vi "ColorMatch_Setting_UI.vi"(0 "Vision_Image In":T3(plugin-control), 1 "Coord?":bool, 5 "List ROI 2":refnum<vi>, 7 "PreProcess In":T1, 9 "ProjectName":string="CDF", 11 "error in (no error)":errorcluster, 12 "Parameter":string, 14 "RootPath":path) -> (4 "Analysis_Setting":string, 6 "Match Flag":bool[](array[boolean]), 8 "Match Score":i32[](array[numeric]), 10 "Cancel?":bool, 15 "error out":errorcluster)   [LabVIEW 2019]
uses:
  <vilib>/vision/NI_Vision_Development_Module.lvlib
  Controls/Analysis_Setting.ctl
  <vilib>/userdefined/High Color/IMAQdx.ctl
  <vilib>/vision/Image Controls.llb/IMAQ Image.ctl
  Controls/_UI Command Cluster/ColorMatch_UI Command.ctl
  Controls/ColorMatch/Analysis_ColorMatch_Parameter.ctl
  cb7ab341-9881-4345-8d5f-fb9cb1b2a84f.vi
  73ae4806-8b8b-4118-bada-9954a96a792c.vi
  <vilib>/Utility/miscctls.llb/LVPointTypeDef.ctl
  c15c5890-f854-46a2-b98b-929fa5ff6ec0.vi
  76c2e7b3-0f24-4336-b544-f46512082401.vi
  Controls/V_Analysis_Type.ctl
  Ctrl/VisionProcessName.ctl
panel:
  out "PreProcess":T1
  in  "Match Saturation Threshold":i32=80 min=10 max=255 step=1
  out "RunROI":T2
  in  "SetROI":bool
  out "TemplateROI":T2
  out "Template Image":T3(plugin-control)
  in  "Cancel":bool
  in  "Done":bool
  in  "ColorMatchTab":T4(tab)
  in  "Minimum Match Score":dbl=750.0 min=10.0 max=255.0 step=1.0
  in  "Color Sensitivity":u32(ring) items=["Low", "Medium", "High"]
  in  "Learn & Match Saturation Threshold":i32=80 min=10 max=255 step=1
  in  "Vision_Image":T3(plugin-control)
  in  "Run Algorithm":bool
  in  "SetTemplate":bool
  # "Use Ctrl to Select multiple ROI"
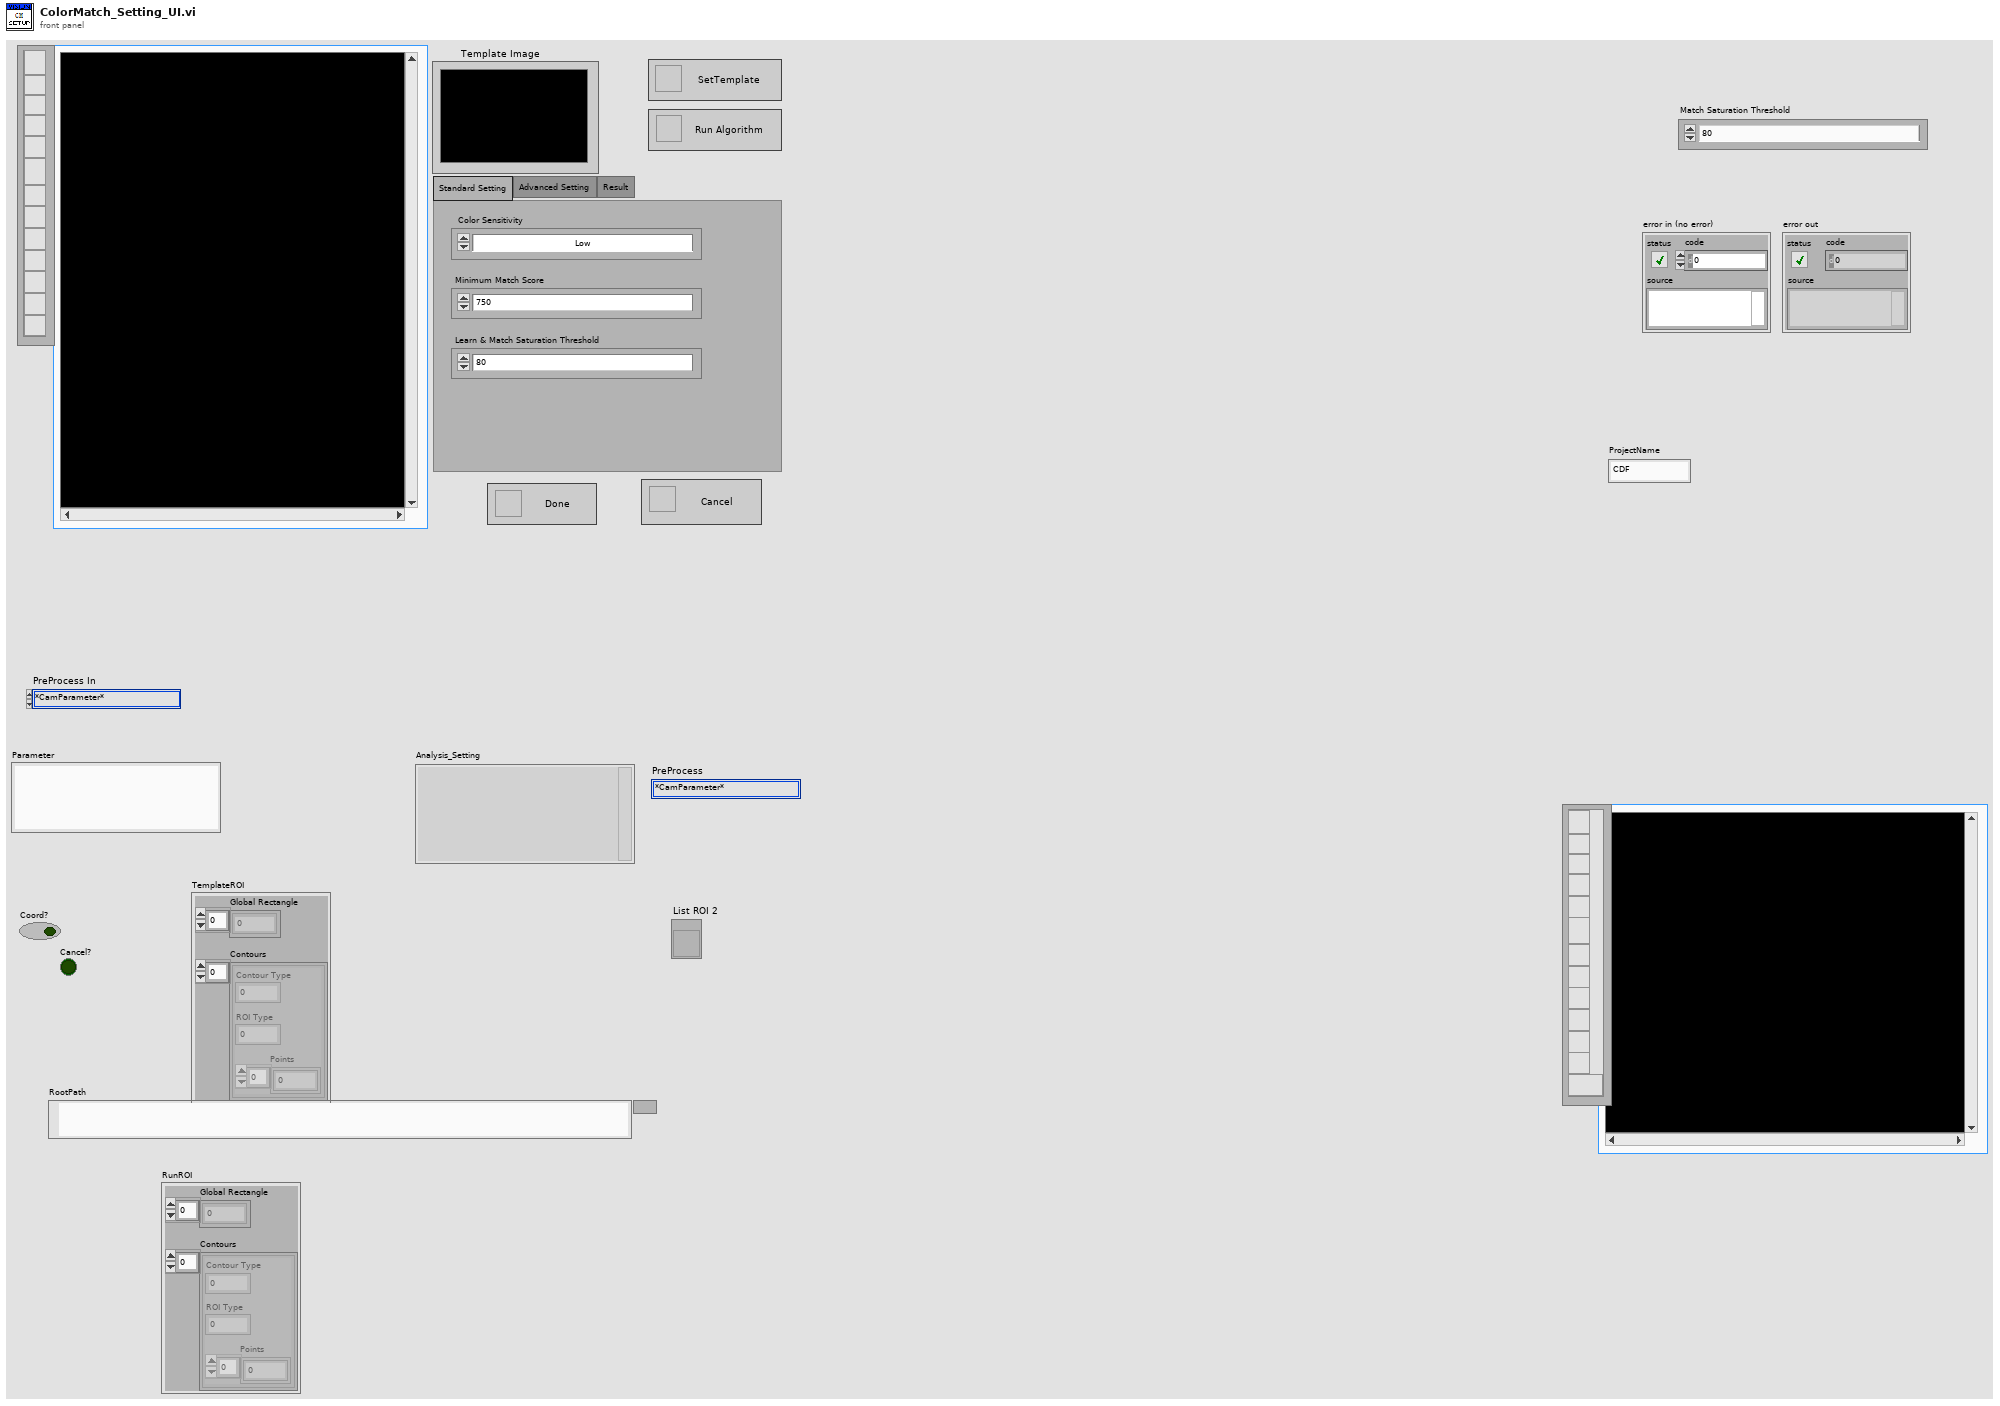
[diagram p1: front panel]
types:
  T1 = typedef "VisionProcessName.ctl" = enum16{"*CamParameter*", "CamAttributes", "*Preprocess*", "CG_Brightness", "C_Plane Extraction", "C_Threshold", "G_Lookup Table", "G_Threshold"}
  T2 = cluster{"Global Rectangle":i32[], "Contours":cluster{"Contour Type":u32, "ROI Type":u32, "Points":i32[]}[]}
  T3 = typedef "IMAQ Image.ctl" = refnum<image>
  T4 = enum32{"Standard Setting", "Advanced Setting", "Result"}
  T5 = typedef "Image Type" = u32
  T6 = typedef "ColorMatch_UI Command.ctl" = enum16{"Init", "Done", "Cancel", "RunAlgorithm", "SetTemplate", "SetROI", "ClearOverlay", "Load Template", "Draw Overlay", "Offset"}
  T7 = typedef "LVPointTypeDef.ctl" = cluster{"Horizontal":i16, "Vertical":i16}
  T8 = typedef "IMAQdx.ctl" = refnum<k21>
  T9 = typedef "Analysis_Setting.ctl" = cluster{"PreProcess":T10, "Parameter":string}
  T10 = typedef "V_Analysis_Type.ctl" = enum16{"None", "C_Color Pattern Matching", "G_PatternMatching", "G_ShapeDectect", "G_GeometricMatch", "B_Area Check"}
  T11 = enum8{"Enabled", "Disabled", "Disabled and Grayed Out"}
  T12 = typedef "Analysis_ColorMatch_Parameter.ctl" = cluster{"Color Sensitivity":u32, "Learn Saturation Threshold":i32, "Minimum Match Score":dbl, "Match Saturation Threshold":i32, "ROI Descriptor":T13, "TemplatePath":string, "ColorSpectrum":dbl[]}
  T13 = typedef "ROI Descriptor" = cluster{"Global Rectangle":i32[], "Contours":cluster{"ID":enum32{"External", "Internal"}, "Type":u32, "Coordinates":i32[]}[]}
  T14 = cluster{"Desired Font (Application)":enum16{"User-specified Font", "Application Font", "System Font", "Dialog Font"}, "[User-specified Font]":cluster{"Font Name":string, "Size":i16, "Strikeout?":bool, "Italic?":bool, "Underline?":bool, "Outline?":bool, "Shadow?":bool, "Bold?":bool, "Rotation Angle":dbl}, "Horizontal Alignment":i16, "Vertical Alignment":i16}
  T15 = cluster{"Contour Type":u32, "ROI Type":u32, "Points":i32[]}
  T16 = cluster{"Position":cluster{"x":sgl, "y":sgl}, "Angle":sgl, "Scale":sgl, "Score":sgl, "Bounding Box":cluster{"x":sgl, "y":sgl}[]}[]
  T17 = cluster{"Contour Type":u32, "ROI Type":u32, "Points":i32[]}[]
  T18 = enum16{"Init", "Done", "Cancel", "RunAlgorithm", "SetTemplate", "SetROI", "ClearOverlay"}
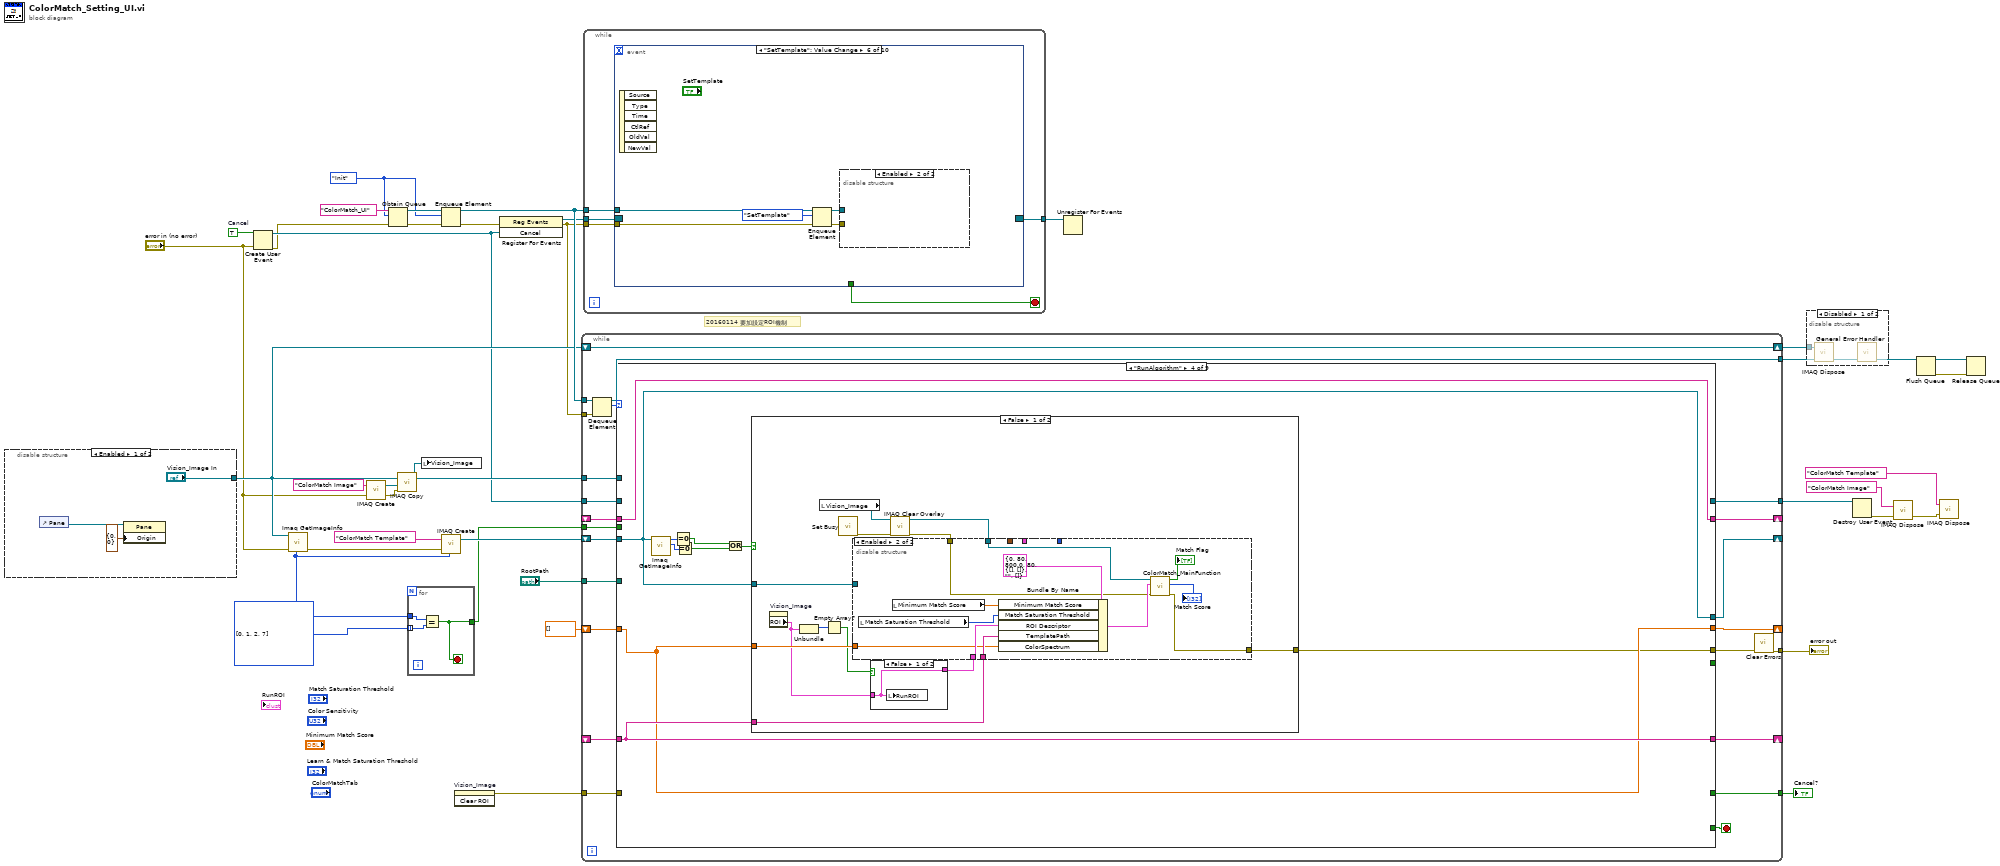
[diagram p0: block diagram]
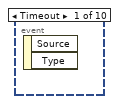
[diagram p2: hidden frame]
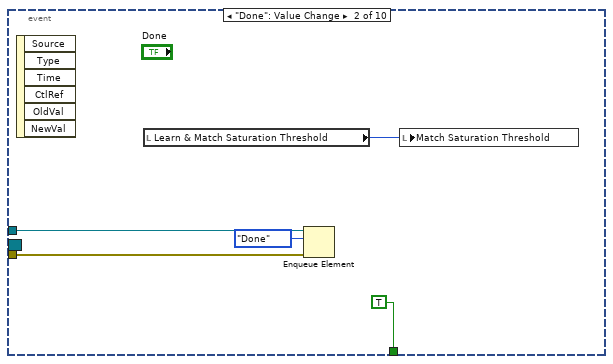
[diagram p3: hidden frame]
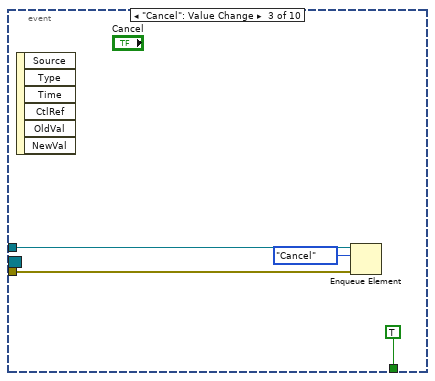
[diagram p4: hidden frame]
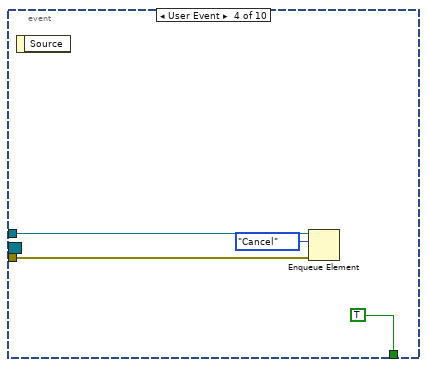
[diagram p5: hidden frame]
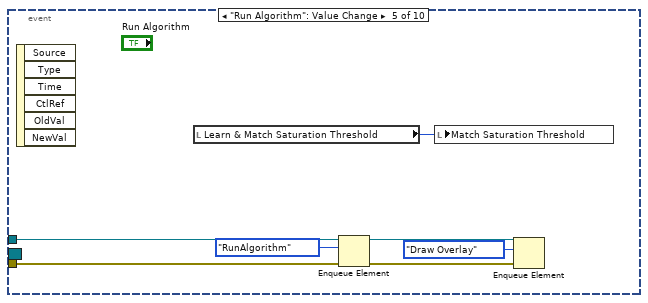
[diagram p6: hidden frame]
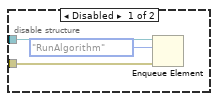
[diagram p7: hidden frame]
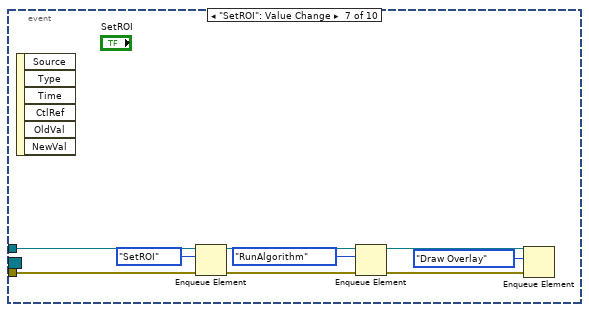
[diagram p8: hidden frame]
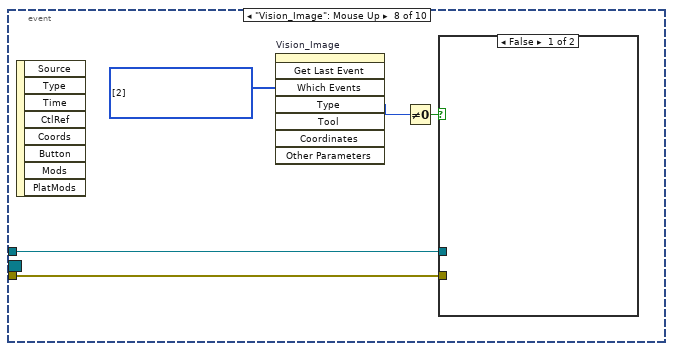
[diagram p9: hidden frame]
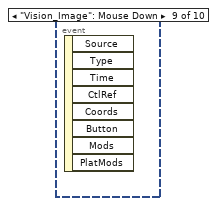
[diagram p11: hidden frame]
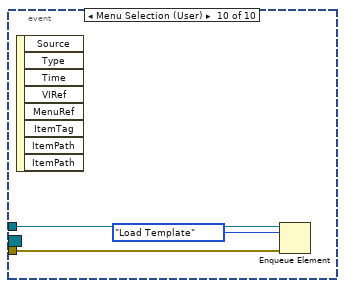
[diagram p12: hidden frame]
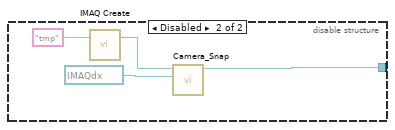
[diagram p13: hidden frame]
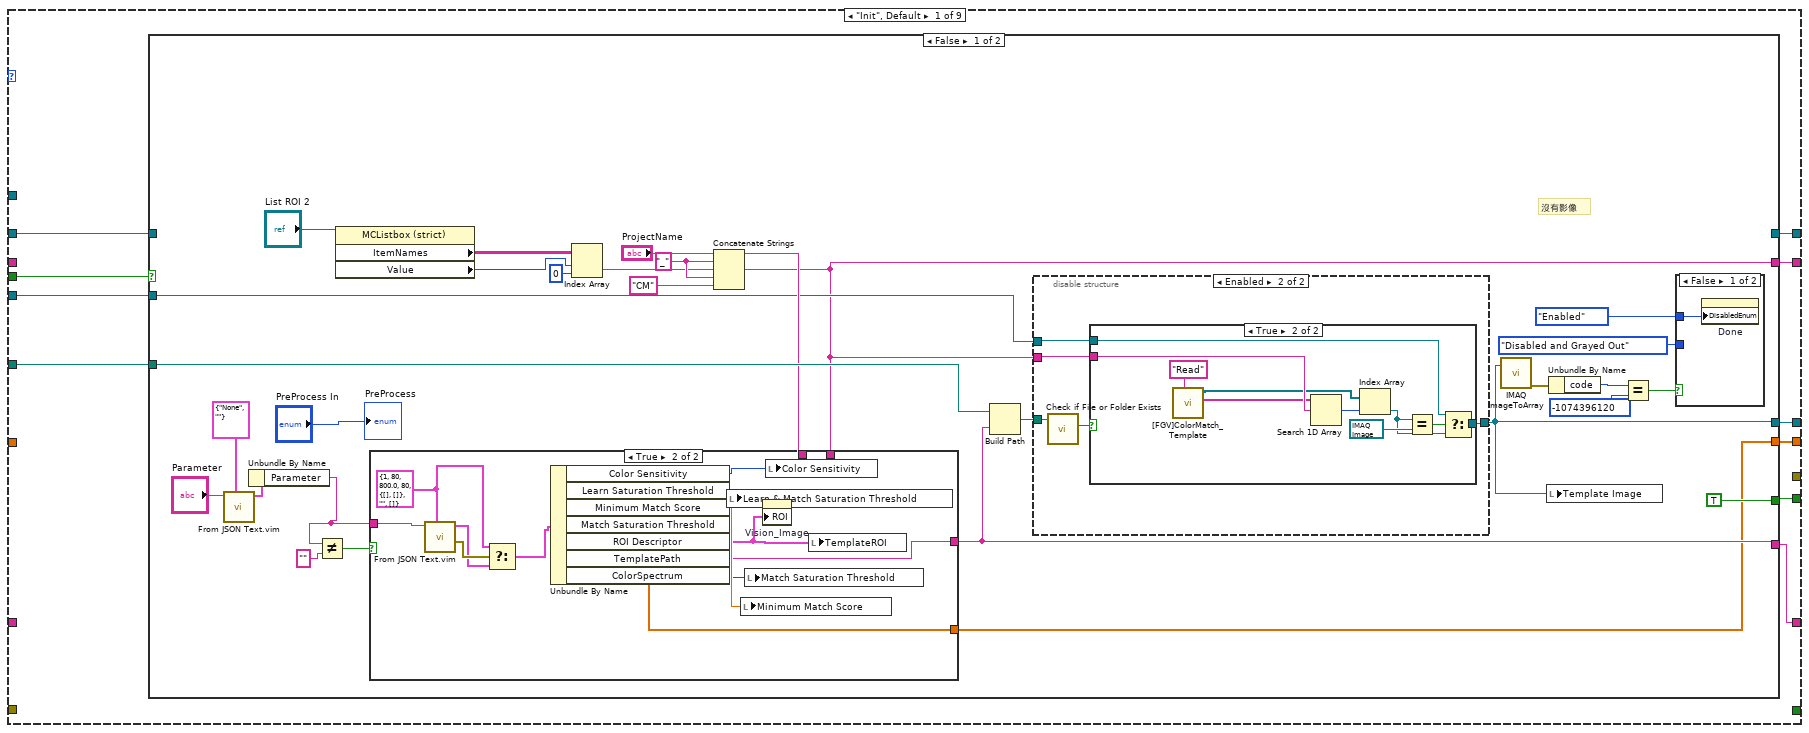
[diagram p15: hidden frame]
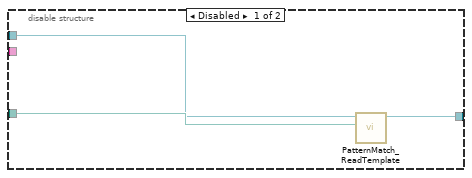
[diagram p16: hidden frame]
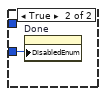
[diagram p18: hidden frame]
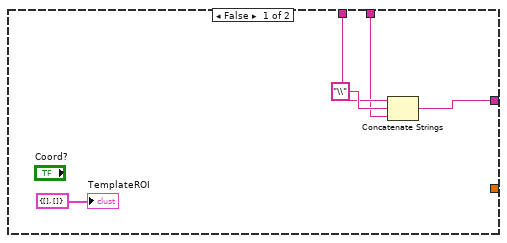
[diagram p19: hidden frame]
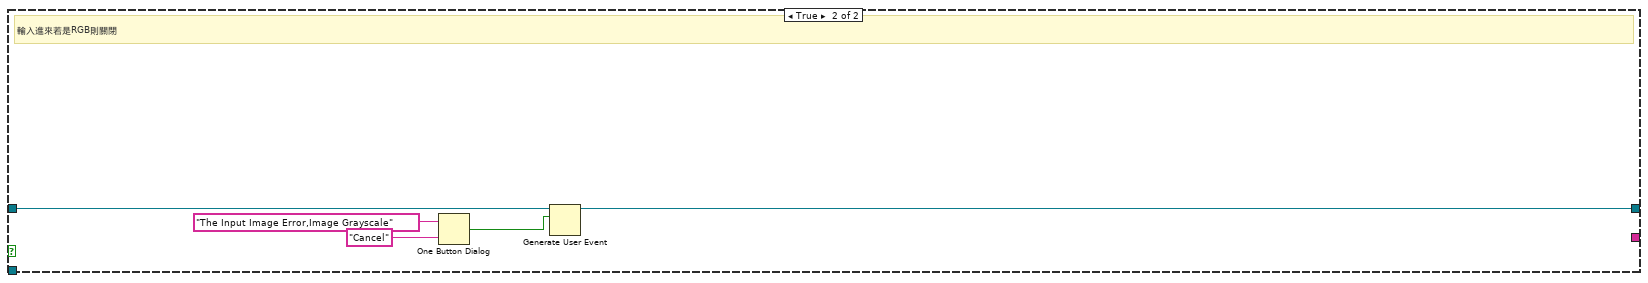
[diagram p20: hidden frame]
diagram:
  w20 = TRUE  # Cancel
  w3 = T5[] [0, 1, 2, 7] items=["Grayscale (U8)", "Grayscale (I16)", "Grayscale (SGL)", "Complex (CSG)", "RGB (U32)", "HSL (U32)", "RGB (U64)", "Grayscale (U16)"] ("x")
  w21 = ColorMatch_UI_Command."Init"
  # "20160114 要加設定ROI機制"
  n1 = disable-structure shown="Enabled" {
    disable-tunnel: ["Vision_Image In" w42] -> w24
    frame Enabled {
      n2 = control-ref of="Pane"() -> (w40:refnum<vi>)
      n3 = property class="Pane"(reference=w40, "Origin"=T7 {"Horizontal"=0, "Vertical"=0}) -> ()  [unwired: 1 in, 2 out]
    }
    frame Disabled {
      n4 = call "IMAQ Create"("Image Name"="tmp") -> ("New Image"=w43:T3)  [unwired: 4 in, 1 out]
      n5 = call "Camera_Snap.vi"("Camera Session In"=T8 "cam0", "Image In"=w43) -> ("New Image"=w42:T3)  [unwired: 8 in, 1 out]
    }
  }
  n6 = Create User Event(user event datatype=w20, error in="error in (no error)") -> (user event=w18:refnum<user-event>, error out=w9:errorcluster)
  n7 = call "Imaq GetImageInfo"("error in (no error)"="error in (no error)", "Image"=w24) -> ("error out"=w7:errorcluster, "Image Type"=w4:T5)  [unwired: 2 in, 6 out]
  n8 = call "IMAQ Create"("Image Name"="ColorMatch Image", "error in (no error)"="error in (no error)") -> ("New Image"=w33:T3, "error out"=w8:errorcluster)  [unwired: 3 in]
  n9 = Obtain Queue(name (unnamed)="ColorMatch_UI", element data type=w21, error in (no error)=w9) -> (queue out=w30:refnum<queue>, error out=w29:errorcluster)  [unwired: 2 in, 1 out]
  n10 = call "IMAQ Copy"("error in (no error)"=w8, "Image Dst"=w33, "Image Src"=w24) -> ("Image Dst Out"=w32:T3)  [unwired: 3 in, 1 out]
  n11 = for {
    tunnel: w4 -> [w48]
    tunnel: w3 -> [w47] mode=indexing
    tunnel: [w46] -> w2
    stop <- w46 stop-if-true
    n12 = Equal?(x=w48, y=w47) -> (x = y?=w46:bool)
  }
  n13 = local write "Vision_Image"(w32) -> ()
  n14 = Enqueue Element(queue=w30, element=w21, error in (no error)=w29) -> (queue out=w26:refnum<queue>, error out=w15:errorcluster)  [unwired: 1 in, 1 out]
  n15 = call "IMAQ Create"("Image Name"="ColorMatch Template", "Image Type"=w4, "error in (no error)"=w7) -> ("New Image"=w23:T3)  [unwired: 2 in, 1 out]
  n16 = invoke on="Vision_Image" class="ImageControl" method="Clear ROI"() -> (error out=w35:errorcluster)  [unwired: 3 in, 2 out]
  n17 = register-events(error in=w15, w18) -> (reference out=w19:refnum<event-registration>, error out=w14:errorcluster)  [unwired: 1 in]
  n18 = while {
    shift-right: [w71] -> w38
    shift-left: w24 -> [w71]
    tunnel: [w67] -> w37
    tunnel: w35 -> [w53]
    tunnel: w32 -> [w70]
    tunnel: w26 -> [w65]
    tunnel: w14 -> [w63]
    tunnel: [w62] -> w25
    shift-right: [w61] -> _
    shift-left: _ -> [w60]
    shift-right: [w58] -> _
    shift-left: w23 -> [w69]
    shift-right: [w59] -> _
    shift-left: _ -> [w68]
    tunnel: "RootPath" -> [w57]
    tunnel: w2 -> [w56]
    tunnel: w18 -> [w55]
    tunnel: [w54] -> w17
    shift-right: [w52] -> _
    shift-left: dbl[] [] ("Color Spectrum") -> [w51]
    tunnel: [w50] -> w1
    stop <- w66 stop-if-true
    n19 = Dequeue Element(queue=w65, error in (no error)=w63) -> (queue out=w62:refnum<queue>, element=w64:T6)  [unwired: 1 in, 2 out]
    n20 = case shown="\"RunAlgorithm\"" w64 {
      tunnel: [_ TRUE w181 _ _ _ _ _ _] -> w66
      tunnel: w70 -> [_ w172 w180 _ w243 _ _ _ _]
      tunnel: w69 -> [w76 _ w179 w186 w245 w282 w334 w345 w360]
      tunnel: [_ _ w181 _ _ _ _ _ _] -> w67
      tunnel: w68 -> [_ w166 w177 w184 w244 w283 w335 w346 w361]
      tunnel: [w80 w171 w178 w191 w246 w284 w336 w347 w362] -> w61
      tunnel: w60 -> [_ w171 w178 w191 w246 w284 w336 w347 w362]
      tunnel: [w78 w166 w177 w184 w244 w283 w335 w346 w361] -> w59
      tunnel: [w81 T3 refnum ("Template Out") T3 refnum ("Template Out") w186 w245 w279 w334 w345 w352] -> w58
      tunnel: [w79 FALSE _ _ _ w281 _ _ _] -> _
      tunnel: w57 -> [w77 _ _ _ _ w280 _ _ w359]
      tunnel: w56 -> [w75 _ _ _ _ _ _ _ _]
      tunnel: w55 -> [w74 w168 w175 _ _ _ _ _ _]
      tunnel: [w73 w168 w175 _ _ _ _ _ _] -> w54
      tunnel: w53 -> [_ _ _ _ w233 _ _ _ _]
      tunnel: [w72 w161 w174 w183 w242 w274 w333 w344 w350] -> w52
      tunnel: w51 -> [_ w161 w174 w183 w242 w273 w333 w344 w350]
      tunnel: [_ _ _ w182 _ _ _ _ _] -> w49
      frame "Init", Default {
        n21 = case shown="False" w75 {
          tunnel: [w101 _] -> w81
          tunnel: [w98 _] -> w80
          tunnel: [TRUE _] -> w79
          tunnel: [w109 _] -> w78
          tunnel: w77 -> [w108 _]
          tunnel: w76 -> [w102 _]
          tunnel: w74 -> [_ w151]
          tunnel: [_ w149] -> w73
          tunnel: [w93 _] -> w72
          frame False {
            w105 = "_" ("string")
            # "沒有影像"
            n22 = call "From JSON Text.vim"("Data Type and Default Value"=T9 {"PreProcess"=enum."None", "Parameter"=""} ("Analysis_Setting In"), "JSON"="Parameter") -> ("Data out"=w85:T9)  [unwired: 8 in, 1 out]
            n23 = Unbundle By Name(w85) -> ("Parameter"=w84:string)
            n24 = Not Equal?(x=w84, y="") -> (x != y?=w87:bool)
            n25 = property class="MCListbox (strict)"(reference="List ROI 2") -> ("ItemNames"=w104:string[][], "Value"=w89:i32)  [unwired: 1 in, 2 out]
            n26 = Index Array(array=w104, index (row)=w89, index (col)=0 ("disabled index (col)")) -> (element=w88:string)
            n27 = Concatenate Strings("ProjectName", w105, w88, w105, "CM" ("string")) -> (w98:string)
            n28 = case shown="True" w87 {
              tunnel: [w132 w137] -> w109
              tunnel: "ProjectName" -> [w134 _]
              tunnel: w84 -> [_ w148]
              tunnel: w98 -> [w133 _]
              tunnel: [_ w142] -> w93
              frame False {
                n29 = Concatenate Strings(w134, "\\" ("string"), w133) -> (w132:string)
                "TemplateROI" <- T2 {"Global Rectangle"=[], "Contours"=[]} ("ROI")
              }
              frame True {
                w138 = T12 {"Color Sensitivity"=1, "Learn Saturation Threshold"=80, "Minimum Match Score"=800.0, "Match Saturation Threshold"=80, "ROI Descriptor"={"Global Rectangle"=[], "Contours"=[]}, "TemplatePath"="", "ColorSpectrum"=[]} ("ColorMatchParameter")
                n30 = call "From JSON Text.vim"("Data Type and Default Value"=w138, "JSON"=w148) -> ("error out"=w141:errorcluster, "Data out"=w139:T12)  [unwired: 8 in]
                n31 = Select(t=w138, s=w141, f=w139) -> (s? t:f=w140:T12)
                n32 = Unbundle By Name(w140) -> ("Color Sensitivity"=w145:u32, "Learn Saturation Threshold"=w146:i32, "Minimum Match Score"=w147:dbl, "Match Saturation Threshold"=w144:i32, "ROI Descriptor"=w143:T13, "TemplatePath"=w137:string, "ColorSpectrum"=w142:dbl[])
                n33 = local write "Learn & Match Saturation Threshold"(w146) -> ()
                n34 = local write "Minimum Match Score"(w147) -> ()
                n35 = local write "Match Saturation Threshold"(w144) -> ()
                n36 = property on="Vision_Image" class="ImageControl"("ROI"=w143) -> ()  [unwired: 2 in, 2 out]
                n37 = local write "Color Sensitivity"(w145) -> ()
                n38 = local write "TemplateROI"(w143) -> ()
              }
            }
            n39 = Build Path(base path=w108, name or relative path=w109) -> (appended path=w103:path)
            n40 = disable-structure shown="Enabled" {
              disable-tunnel: w103 -> [w113 w117]
              disable-tunnel: w102 -> [w112 w114]
              disable-tunnel: [w111 w115] -> w101
              disable-tunnel: w98 -> [_ w118]
              frame Disabled {
                n41 = call "PatternMatch_ReadTemplate.vi"("template path"=w113, "Template"=w112) -> ("Template Out"=w111:T3)  [unwired: 8 in, 1 out]
              }
              frame Enabled {
                n42 = call <vilib>:"Check if File or Folder Exists.vi"("path"=w117) -> ("file or folder exists?"=w116:bool)  [unwired: 8 in, 2 out]
                n43 = case shown="True" w116 {
                  tunnel: w118 -> [_ w129]
                  tunnel: [w119 w123] -> w115
                  tunnel: w114 -> [w119 w125]
                  frame False {
                  }
                  frame True {
                    n44 = call "[FGV]ColorMatch_Template.vi"("CMTemplateCommand"="Read") -> ("Image Name Array 2"=w120:string[], "Image Array 2"=w121:T3[])  [unwired: 8 in, 1 out]
                    n45 = Search 1D Array(1D array=w120, element=w129) -> (index of element=w128:i32)  [unwired: 1 in]
                    n46 = Index Array(array=w121, index=w128) -> (element=w124:T3)
                    n47 = Equal?(x=w124, y=T3 refnum) -> (x = y?=w126:bool)
                    n48 = Select(t=w125, s=w126, f=w124) -> (s? t:f=w123:T3)
                  }
                }
              }
            }
            n49 = call "IMAQ ImageToArray"("Image"=w101) -> ("error out"=w97:errorcluster)  [unwired: 3 in, 4 out]
            n50 = local write "Template Image"(w101) -> ()
            n51 = Unbundle By Name(w97) -> ("code"=w96:i32)
            n52 = Equal?(x=w96, y=-1074396120) -> (x = y?=w94:bool)
            n53 = case shown="False" w94 {
              tunnel: T11."Disabled and Grayed Out" ("Disabled") -> [_ w131]
              tunnel: T11."Enabled" ("Disabled") -> [w130 _]
              frame False {
                n54 = property on="Done" class="Bool"("DisabledEnum"=w130) -> ()  [unwired: 2 in, 2 out]
              }
              frame True {
                n55 = property on="Done" class="Bool"("DisabledEnum"=w131) -> ()  [unwired: 2 in, 2 out]
              }
            }
            "PreProcess" <- "PreProcess In"
          }
          frame True {
            # "輸入進來若是RGB則關閉"
            n56 = One Button Dialog(message="The Input Image Error,Image Grayscale", button name ("OK")="Cancel") -> (true=w150:bool)
            n57 = Generate User Event(user event=w151, event data cluster=w150) -> (user event out=w149:refnum<user-event>)  [unwired: 2 in, 1 out]
          }
        }
      }
      frame "Done" {
        w158 = T9 {"PreProcess"=enum."None", "Parameter"=""}  # Analysis_Setting
        (unwired) T15 {"Contour Type"=0, "ROI Type"=0, "Points"=[]} ("RegionContour")
        n58 = local read "Match Saturation Threshold"() -> (w162:i32)
        n59 = local read "Learn & Match Saturation Threshold"() -> (w164:i32)
        n60 = call "IMAQ Dispose"("Image"=w172) -> ()  [unwired: 5 in, 1 out]
        n61 = local read "RunROI"() -> (w160:T2)
        n62 = local read "Color Sensitivity"() -> (w163:u32)
        n63 = local read "Minimum Match Score"() -> (w165:dbl)
        n64 = Bundle By Name(cluster=T12 {"Color Sensitivity"=0, "Learn Saturation Threshold"=80, "Minimum Match Score"=800.0, "Match Saturation Threshold"=80, "ROI Descriptor"={"Global Rectangle"=[], "Contours"=[]}, "TemplatePath"="", "ColorSpectrum"=[]} ("ColorMatchParameter"), "Color Sensitivity"=w163, "Learn Saturation Threshold"=w164, "Minimum Match Score"=w165, "Match Saturation Threshold"=w162, "ROI Descriptor"=w160, "TemplatePath"=w166, "ColorSpectrum"=w161) -> (w159:T12)
        n65 = call "To JSON Text.vim"("Anything"=w159) -> ("<JSON>"=w157:string)  [unwired: 9 in, 1 out]
        n66 = local read "PreProcess"() -> (w154:T1)
        n67 = Bundle(cluster=w158, "PreProcess"=w154, "Parameter"=w157) -> (w156:T9)
        n68 = call "To JSON Text.vim"("Anything"=w156) -> ("<JSON>"=→"Analysis_Setting":string)  [unwired: 9 in, 1 out]
      }
      frame "Cancel" {
        w181 = TRUE
        n69 = call "IMAQ Dispose"("Image"=w179) -> ()  [unwired: 5 in, 1 out]
        n70 = call "IMAQ Dispose"("Image"=w180) -> ()  [unwired: 5 in, 1 out]
      }
      frame "RunAlgorithm" {
        n71 = call "Imaq GetImageInfo"("Image"=w186) -> ("Y Resolution"=w190:i32, "X Resolution"=w189:i32)  [unwired: 3 in, 6 out]
        n72 = Equal To 0?(x=w189) -> (x = 0?=w188:bool)
        n73 = Equal To 0?(x=w190) -> (x = 0?=w187:bool)
        n74 = Or(x=w188, y=w187) -> (x .or. y?=w185:bool)
        n75 = case shown="False" w185 {
          tunnel: w186 -> [w199 _]
          tunnel: w184 -> [w198 _]
          tunnel: w183 -> [w197 _]
          tunnel: [w196 _] -> w182
          frame False {
            n76 = property on="Vision_Image" class="ImageControl"() -> ("ROI"=w192:T2)  [unwired: 2 in, 2 out]
            n77 = Unbundle(w192) -> ("Global Rectangle"=w194:i32[])  [unwired: 1 out]
            n78 = local read "Vision_Image"() -> (w200:T3)
            n79 = Empty Array?(array=w194) -> (empty?=w193:bool)
            n80 = call <vilib>:"Set Busy.vi"() -> ("error out"=w203:errorcluster)  [unwired: 10 in, 1 out]
            n81 = case shown="False" w193 {
              tunnel: [w204 w205] -> w195
              tunnel: w192 -> [w204 _]
              frame False {
                n82 = local write "RunROI"(w204) -> ()
              }
              frame True {
                n83 = local read "RunROI"() -> (w205:T2)
              }
            }
            n84 = call "IMAQ Clear Overlay"("error in (no error)"=w203, "Image"=w200) -> ("error out"=w201:errorcluster, "Image Out"=w202:T3)  [unwired: 8 in]
            n85 = disable-structure shown="Enabled" {
              disable-tunnel: w199 -> [w215 _]
              disable-tunnel: w201 -> [w214 w224]
              disable-tunnel: _ -> [w212 _]
              disable-tunnel: _ -> [w211 _]
              disable-tunnel: _ -> [w210 _]
              disable-tunnel: w202 -> [w209 w228]
              disable-tunnel: w195 -> [w206 w223]
              disable-tunnel: w198 -> [_ w222]
              disable-tunnel: w197 -> [_ w221]
              disable-tunnel: [_ w218] -> w196
              frame Disabled {
                w217 = 0 items=["All", "Low Discrepancy Sampling", "Grayscale Value Pyramid", "Gradients Pyramid"] ("Algorithm")
                n86 = call "IMAQ Learn Pattern 4"("Algorithm"=w217, "error in (no error)"=w214, "Angle Range"=cluster{"Start Angle":sgl, "End Angle":sgl} {"Start Angle"=0.0, "End Angle"=360.0}, "Image"=w215) -> ("error out"=w213:errorcluster, "Template Image Out"=w207:T3)  [unwired: 5 in, 1 out]
                n87 = call "IMAQ Match Pattern 4"("Image"=w209, "Algorithm"=w211, "Template Image"=w207, "ROI Descriptor"=w206, "Parameters"=w212, "error in (no error)"=w213, "Advanced Options"=w210) -> ("Matches (pixel)"=w208:T16)  [unwired: 4 in, 4 out]
              }
              frame Enabled {
                n88 = local read "Match Saturation Threshold"() -> (w219:i32)
                n89 = local read "Minimum Match Score"() -> (w220:dbl)
                n90 = Bundle By Name(cluster=T12 {"Color Sensitivity"=0, "Learn Saturation Threshold"=80, "Minimum Match Score"=800.0, "Match Saturation Threshold"=80, "ROI Descriptor"={"Global Rectangle"=[], "Contours"=[]}, "TemplatePath"="", "ColorSpectrum"=[]} ("ColorMatchParameter"), "Minimum Match Score"=w220, "Match Saturation Threshold"=w219, "ROI Descriptor"=w223, "TemplatePath"=w222, "ColorSpectrum"=w221) -> (w227:T12)
                n91 = call "ColorMatch_MainFunction.vi"("error in (no error)"=w224, "ColorMatchParameter"=w227, "Vision_Image In"=w228) -> ("error out"=w218:errorcluster, "Match Score"=→"Match Score":i32[], "Match Flag"=→"Match Flag":bool[])  [unwired: 6 in]
              }
            }
          }
          frame True {
            n92 = One Button Dialog(message="No Template is Set~!!!\nPlease Set Template Before Analyze~!!") -> ()  [unwired: 1 in, 1 out]
          }
        }
      }
      frame "Draw Overlay" {
        n93 = invoke on="Vision_Image" class="ImageControl" method="Clear ROI"(error in=w233) -> (error out=w232:errorcluster)  [unwired: 2 in, 2 out]
        n94 = call "IMAQ Clear Overlay"("error in (no error)"=w232, "Image"=w243) -> ("error out"=w241:errorcluster, "Image Out"=w236:T3)  [unwired: 8 in]
        n95 = local read "RunROI"() -> (w235:T2)
        n96 = local read "Match Flag"() -> (w239:bool[])
        n97 = call "IMAQ Overlay ROI"("Colors (Green)"=u32[] [16776770], "ROI Descriptor"=w235, "Image"=w236) -> ("Image Out"=w234:T3)  [unwired: 7 in, 1 out]
        n98 = Unbundle(w235) -> ("Contours"=w237:T17)  [unwired: 1 out]
        n99 = for {
          shift-right: [w250] -> w240
          shift-left: w241 -> [w251]
          shift-right: [w249] -> w238
          shift-left: w234 -> [w252]
          tunnel: w239 -> [w248] mode=indexing
          tunnel: w237 -> [w247] mode=indexing
          n100 = case shown="True" w248 {
            tunnel: w252 -> [w257 w266]
            tunnel: w247 -> [w254 w269]
            tunnel: w251 -> [w256 w265]
            tunnel: [w260 w270] -> w249
            tunnel: [w255 w264] -> w250
            frame False {
              # "Use first two coordinates of ROI to make point"
              n101 = Unbundle By Name(w254) -> ("Points"=w253:i32[])
              n102 = Array To Cluster(array=w253) -> (cluster=w259:cluster{"Points[0]":i32, "Points[1]":i32})
              n103 = call "IMAQ Overlay Text"("BG Color (Transparent)"=u32 16711680, "Font, Size & Style"=T14 {"Desired Font (Application)"=enum."Application Font", "[User-specified Font]"={"Font Name"="", "Size"=12, "Strikeout?"=FALSE, "Italic?"=FALSE, "Underline?"=FALSE, "Outline?"=FALSE, "Shadow?"=FALSE, "Bold?"=FALSE, "Rotation Angle"=0.0}, "Horizontal Alignment"=0, "Vertical Alignment"=1}, "error in (no error)"=w256, "String"="FAIL", "Origin"=w259, "Image"=w257) -> ("error out"=w255:errorcluster, "Image Out"=w260:T3)  [unwired: 4 in]
            }
            frame True {
              # "Use first two coordinates of ROI to make point"
              n104 = Unbundle By Name(w269) -> ("Points"=w263:i32[])
              n105 = Array To Cluster(array=w263) -> (cluster=w268:cluster{"Points[0]":i32, "Points[1]":i32})
              n106 = call "IMAQ Overlay Text"("BG Color (Transparent)"=u32 6618880, "Font, Size & Style"=T14 {"Desired Font (Application)"=enum."Application Font", "[User-specified Font]"={"Font Name"="", "Size"=12, "Strikeout?"=FALSE, "Italic?"=FALSE, "Underline?"=FALSE, "Outline?"=FALSE, "Shadow?"=FALSE, "Bold?"=FALSE, "Rotation Angle"=0.0}, "Horizontal Alignment"=0, "Vertical Alignment"=1}, "error in (no error)"=w265, "String"="PASS", "Origin"=w268, "Image"=w266) -> ("error out"=w264:errorcluster, "Image Out"=w270:T3)  [unwired: 4 in]
            }
          }
        }
        n107 = local write "Vision_Image"(w238) -> ()
        n108 = call <vilib>:"Unset Busy.vi"("error in (no error)"=w240) -> ()  [unwired: 10 in, 1 out]
      }
      frame "SetTemplate" {
        # "沒有影像"
        # "-1074396120"
        n109 = call "Imaq GetImageInfo"("Image"=w282) -> ("error out"=w278:errorcluster)  [unwired: 3 in, 7 out]
        n110 = Unbundle By Name(w278) -> ("code"=w277:i32)
        n111 = Equal?(x=w277, y=-1074396120) -> (x = y?=w275:bool)
        n112 = case shown="True" w275 {
          tunnel: [w287 TRUE] -> w285
          frame False {
            n113 = Two Button Dialog(message="Template Already Exist, You Sure to Create New Template?") -> (T button?=w287:bool)  [unwired: 2 in]
          }
          frame True {
          }
        }
        n114 = case shown="True" w285 {
          tunnel: w282 -> [w290 w298]
          tunnel: w283 -> [_ w297]
          tunnel: [_ w296] -> w281
          tunnel: w280 -> [_ w295]
          tunnel: [w290 w294] -> w279
          tunnel: [w289 w293] -> w274
          tunnel: w273 -> [w289 w292]
          frame False {
          }
          frame True {
            n115 = property on="Vision_Image" class="ImageControl"() -> ("ROI"=w291:T2)  [unwired: 2 in, 2 out]
            n116 = Unbundle By Name(w291) -> ("Contours"=w302:T17, "Global Rectangle"=w299:i32[])
            n117 = local write "TemplateROI"(w291) -> ()
            n118 = Array Size(array=w302) -> (size(s)=w301:i32)
            n119 = Not Equal To 0?(x=w301) -> (x != 0?=w300:bool)
            n120 = case shown="True" w300 {
              tunnel: w299 -> [_ w322]
              tunnel: w298 -> [w304 w321]
              tunnel: w297 -> [_ w317]
              tunnel: [_ TRUE] -> w296
              tunnel: w295 -> [_ w318]
              tunnel: [w304 w307] -> w294
              tunnel: [w303 w309] -> w293
              tunnel: w292 -> [w303 _]
              frame False {
                n121 = One Button Dialog(message="Please Select Template On the Image") -> ()  [unwired: 1 in, 1 out]
              }
              frame True {
                n122 = local read "Learn & Match Saturation Threshold"() -> (w311:i32)
                n123 = call <vilib>:"Set Busy.vi"() -> ("error out"=w314:errorcluster)  [unwired: 10 in, 1 out]
                n124 = local read "Color Sensitivity"() -> (w312:u32)
                n125 = Build Path(base path=w318, name or relative path=w317) -> (appended path=w316:path)
                n126 = call "IMAQ Extract"("Optional Rectangle"=w322, "error in (no error)"=w314, "Image Dst"=w321, "Image Src"="Vision_Image") -> ("error out"=w315:errorcluster, "Image Dst Out"=w313:T3)  [unwired: 6 in]
                n127 = call "IMAQ ColorLearn"("Image"=w313, "Color Sensitivity"=w312, "Learn Saturation Threshold"=w311) -> ("Color Spectrum"=w308:dbl[], "error out"=w310:errorcluster)  [unwired: 5 in]
                n128 = invoke on="Vision_Image" class="ImageControl" method="Clear ROI"(error in=w315) -> ()  [unwired: 2 in, 3 out]
                n129 = case shown="No Error" w310 {
                  tunnel: w316 -> [w328 _]
                  tunnel: w313 -> [w324 _]
                  tunnel: [w323 T3 refnum ("Image Dst Out")] -> w307
                  tunnel: [w326 w329] -> w309
                  tunnel: w308 -> [w326 w329]
                  tunnel: [w325 _] -> w306
                  frame No Error {
                    n130 = property on="Done" class="Bool"("DisabledEnum"=T11."Enabled" ("Disabled")) -> ()  [unwired: 2 in, 2 out]
                    n131 = call-poly "IMAQ Write File 2"("File Path"=w328, "Image"=w324) -> ("error out"=w325:errorcluster, "Image Out (duplicate)"=w323:T3)  [unwired: 8 in]
                  }
                  frame Error {
                    n132 = One Button Dialog(message="Invalid learn setup data.\nplease Reset Set", button name ("OK")="OK") -> ()  [unwired: 1 out]
                  }
                }
                "Template Image" <- w307
                n133 = call <vilib>:"Unset Busy.vi"("error in (no error)"=w306) -> ()  [unwired: 10 in, 1 out]
              }
            }
          }
        }
      }
      frame "SetROI" {
        n134 = property on="Vision_Image" class="ImageControl"() -> ("ROI"=w337:T2)  [unwired: 2 in, 2 out]
        n135 = Unbundle By Name(w337) -> ("Global Rectangle"=w339:i32[])
        n136 = Array Size(array=w339) -> (size(s)=w340:i32)
        n137 = Not Equal To 0?(x=w340) -> (x != 0?=w338:bool)
        n138 = case shown="True" w338 {
          tunnel: w337 -> [_ w342]
          frame False {
            n139 = One Button Dialog(message="Please Select An Area As ROI") -> ()  [unwired: 1 in, 1 out]
          }
          frame True {
            n140 = disable-structure shown="Enabled" {
              disable-tunnel: w342 -> [w343 _]
              frame Enabled {
                n141 = local write "TemplateROI"(w343) -> ()
              }
              frame Disabled {
              }
            }
          }
        }
      }
      frame "ClearOverlay" {
        n142 = local read "Vision_Image"() -> (w349:T3)
        n143 = call "IMAQ Clear Overlay"("Image"=w349) -> ("Image Out"=w348:T3)  [unwired: 9 in, 1 out]
        n144 = local write "Vision_Image"(w348) -> ()
      }
      frame "Load Template" {
        # "這個不需要改，因為這是開放給使用者自己去選的"
        # "後面不需要去做Learn Pattern的動作，因為讀進的Pattern都是已經Learn過"
        n145 = Build Path(base path=w359, name or relative path="\\Data") -> (appended path=w358:path)
        n146 = call "File Dialog"("start path"=w358) -> ("selected path"=w357:path, "cancelled"=w356:bool, "error out"=w355:errorcluster)  [unwired: 11 in, 1 out]
        n147 = call <vilib>:"Clear Errors.vi"("error in (no error)"=w355) -> ()  [unwired: 5 in, 2 out]
        n148 = case shown="False" w356 {
          tunnel: w360 -> [w366 w367]
          tunnel: [w365 w367] -> w352
          tunnel: w357 -> [w364 _]
          frame False {
            n149 = call "PatternMatch_ReadTemplate.vi"("template path"=w364, "Template"=w366) -> ("Template Out"=w365:T3)  [unwired: 8 in, 1 out]
          }
          frame True {
          }
        }
        n150 = local write "Template Image"(w352) -> ()
        n151 = call "IMAQ ImageToArray"("Image"=w352) -> ("Image Pixels (U8)"=w353:u8[][])  [unwired: 3 in, 4 out]
        n152 = Empty Array?(array=w353) -> (empty?=w351:bool)
        n153 = case shown="False" w351 {
          frame False {
            n154 = property on="Done" class="Bool"("DisabledEnum"=T11."Enabled" ("Disabled")) -> ()  [unwired: 2 in, 2 out]
          }
          frame True {
          }
        }
      }
    }
    n155 = call <vilib>:"Clear Errors.vi"("error in (no error)"=w49) -> ("error out"=w50:errorcluster)  [unwired: 5 in, 1 out]
  }
  "error out" <- w1
  "Cancel?" <- w37
  n156 = while {
    tunnel: w26 -> [w371]
    tunnel: w14 -> [w370]
    tunnel: w19 -> [w369]
    tunnel: [w368] -> w16
    stop <- w372 stop-if-true
    n157 = event shown="[5] \"SetTemplate\": Value Change" {
      selector: w369 -> [_ _ _ _ _ _ _ _ _ _]
      dyn-events: [_ _ _ _ _ _ _ _ _ _] -> w368
      timeout: _ -> [_ _ _ _ _ _ _ _ _ _]
      tunnel: [_ TRUE TRUE TRUE _ _ _ _ _ _] -> w372
      tunnel: w371 -> [_ w376 w380 w384 w392 w397 w409 w411 _ w417]
      tunnel: w370 -> [_ w375 w379 w383 w391 w396 w408 w410 _ w416]
      event Timeout {
        n158 = event-data() -> ()  [unwired: 1 in, 2 out]
      }
      event "Done": Value Change {
        n159 = event-data() -> ()  [unwired: 1 in, 6 out]
        n160 = local read "Learn & Match Saturation Threshold"() -> (w373:i32)
        n161 = Enqueue Element(queue=w376, element=ColorMatch_UI_Command."Done", error in (no error)=w375) -> ()  [unwired: 1 in, 3 out]
        n162 = local write "Match Saturation Threshold"(w373) -> ()
      }
      event "Cancel": Value Change {
        n163 = event-data() -> ()  [unwired: 1 in, 6 out]
        n164 = Enqueue Element(queue=w380, element=ColorMatch_UI_Command."Cancel", error in (no error)=w379) -> ()  [unwired: 1 in, 3 out]
      }
      event User Event {
        n165 = event-data() -> ()  [unwired: 1 in, 1 out]
        n166 = Enqueue Element(queue=w384, element=ColorMatch_UI_Command."Cancel", error in (no error)=w383) -> ()  [unwired: 1 in, 3 out]
      }
      event "Run Algorithm": Value Change {
        n167 = event-data() -> ()  [unwired: 1 in, 6 out]
        n168 = local read "Learn & Match Saturation Threshold"() -> (w386:i32)
        n169 = Enqueue Element(queue=w392, element=ColorMatch_UI_Command."RunAlgorithm", error in (no error)=w391) -> (queue out=w388:refnum<queue>, error out=w389:errorcluster)  [unwired: 1 in, 1 out]
        n170 = local write "Match Saturation Threshold"(w386) -> ()
        n171 = Enqueue Element(queue=w388, element=ColorMatch_UI_Command."Draw Overlay", error in (no error)=w389) -> ()  [unwired: 1 in, 3 out]
      }
      event "SetTemplate": Value Change {
        n172 = event-data() -> ()  [unwired: 1 in, 6 out]
        n173 = Enqueue Element(queue=w397, element=ColorMatch_UI_Command."SetTemplate", error in (no error)=w396) -> (queue out=w394:refnum<queue>, error out=w393:errorcluster)  [unwired: 1 in, 1 out]
        n174 = disable-structure shown="Enabled" {
          disable-tunnel: w394 -> [w400 _]
          disable-tunnel: w393 -> [w399 _]
          frame Disabled {
            n175 = Enqueue Element(queue=w400, element=T18."RunAlgorithm", error in (no error)=w399) -> ()  [unwired: 1 in, 3 out]
          }
          frame Enabled {
          }
        }
      }
      event "SetROI": Value Change {
        n176 = event-data() -> ()  [unwired: 1 in, 6 out]
        n177 = Enqueue Element(queue=w409, element=ColorMatch_UI_Command."SetROI", error in (no error)=w408) -> (queue out=w406:refnum<queue>, error out=w405:errorcluster)  [unwired: 1 in, 1 out]
        n178 = Enqueue Element(queue=w406, element=ColorMatch_UI_Command."RunAlgorithm", error in (no error)=w405) -> (queue out=w402:refnum<queue>, error out=w403:errorcluster)  [unwired: 1 in, 1 out]
        n179 = Enqueue Element(queue=w402, element=ColorMatch_UI_Command."Draw Overlay", error in (no error)=w403) -> ()  [unwired: 1 in, 3 out]
      }
      event "Vision_Image": Mouse Up {
        w412 = i32[] [2] items=["No Event"=0, "Click Event"=1, "Draw Event"=2, "Size Event"=4, "Scroll Event"=5, "Double Click Event"=8] ("Which Events")
        n180 = event-data() -> ()  [unwired: 1 in, 8 out]
        n181 = invoke on="Vision_Image" class="ImageControl" method="Get Last Event"("Which Events"=w412) -> ("Type"=w413:i32)  [unwired: 7 in, 7 out]
        n182 = Not Equal To 0?(x=w413) -> (x != 0?=w414:bool)
        n183 = case shown="False" w414 {
          tunnel: w411 -> [_ _]
          tunnel: w410 -> [_ _]
          frame False {
          }
          frame True {
          }
        }
      }
      event "Vision_Image": Mouse Down {
        n184 = event-data() -> ()  [unwired: 1 in, 8 out]
      }
      event Menu Selection (User) {
        n185 = event-data() -> ()  [unwired: 1 in, 8 out]
        n186 = Enqueue Element(queue=w417, element=ColorMatch_UI_Command."Load Template", error in (no error)=w416) -> ()  [unwired: 1 in, 3 out]
      }
    }
  }
  n187 = Unregister For Events(event registration refnum=w16) -> ()  [unwired: 1 in, 1 out]
  n188 = disable-structure shown="Disabled" {
    disable-tunnel: w38 -> [w418 _]
    frame Disabled {
      n189 = call "IMAQ Dispose"("Image"=w418) -> ("error out"=w419:errorcluster)  [unwired: 5 in]
      n190 = call <vilib>:"General Error Handler.vi"("error in (no error)"=w419) -> ()  [unwired: 2 in, 13 out]
    }
    frame Enabled {
    }
  }
  n191 = Destroy User Event(user event=w17) -> (error out=w13:errorcluster)  [unwired: 1 in]
  n192 = call "IMAQ Dispose"("Image"="ColorMatch Image" ("Image Name"), "error in (no error)"=w13) -> ("error out"=w11:errorcluster)  [unwired: 4 in]
  n193 = Flush Queue(queue=w25) -> (queue out=w28:refnum<queue>, error out=w27:errorcluster)  [unwired: 1 in, 1 out]
  n194 = call "IMAQ Dispose"("Image"="ColorMatch Template" ("Image Name"), "error in (no error)"=w11) -> ()  [unwired: 4 in, 1 out]
  n195 = Release Queue(queue=w28, error in (no error)=w27) -> ()  [unwired: 1 in, 3 out]
